vi "בדיקת זמן מיתוג הממסר 6.vi"(8 "error":errorcluster, 11 "Path for Log":path) -> (0 "error out":errorcluster, 1 "בטוח כן/לא":bool, 2 "בדיקת זמן מיתוג הממסר":dbl, 7 "Userresult":bool)   [LabVIEW 2014]
uses:
  <instrlib>/niDMM/nidmm.llb/niDMM Function.ctl
  <instrlib>/niDMM/nidmm.llb/niDMM Resolution in Digits.ctl
  <vilib>/DAQmx/create/channels.llb/DAQmx Create Channel (DO-Digital Output).vi
  <instrlib>/niDMM/nidmm.llb/niDMM Configure Measurement Digits.vi
  <vilib>/DAQmx/write.llb/DAQmx Write (Digital Bool 1Line 1Point).vi
panel:
  in  "התחל":bool
  # "Right-Click to\nexplain error"
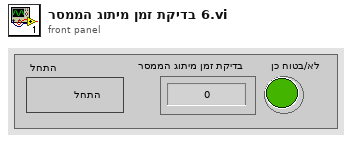
[diagram p1: front panel]
types:
  T1 = enum32{"Invalid", "Standard", "Closed", "Hidden", "Minimized", "Maximized"}
  T2 = typedef "niDMM Function.ctl" = enum16{"DC Volts", "AC Volts", "DC Current", "AC Current", "2-wire Resistance", "4-wire Resistance", "Diode", "Frequency", "Period", "AC Volts DC Coupled", "Capacitance", "Inductance", "Temperature"}
  T3 = typedef "niDMM Resolution in Digits.ctl" = dbl
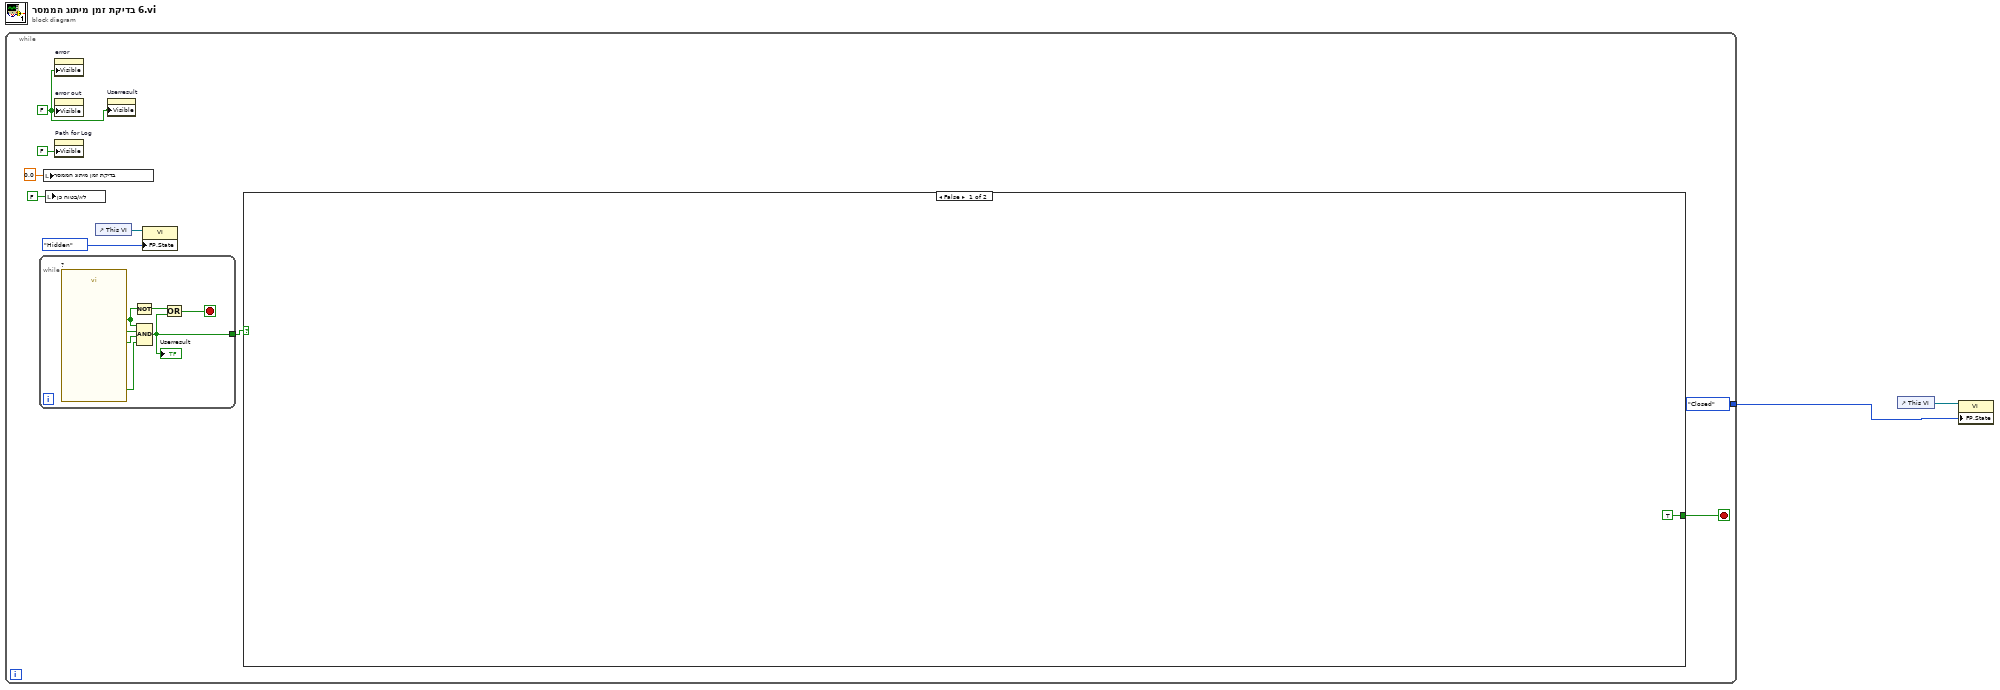
[diagram p0: block diagram]
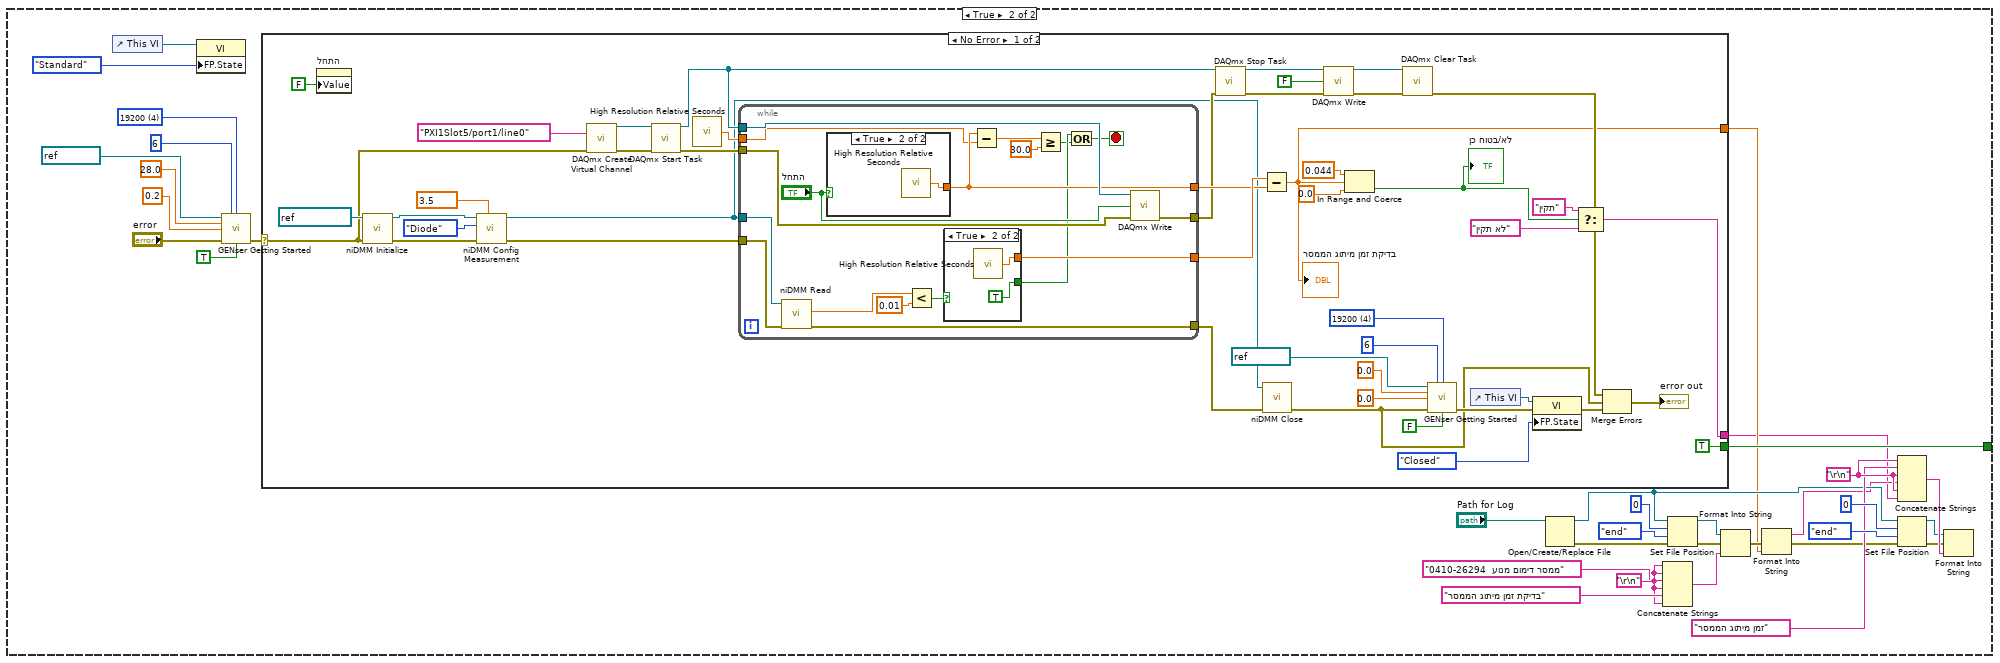
[diagram p2: hidden frame]
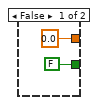
[diagram p3: hidden frame]
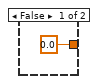
[diagram p4: hidden frame]
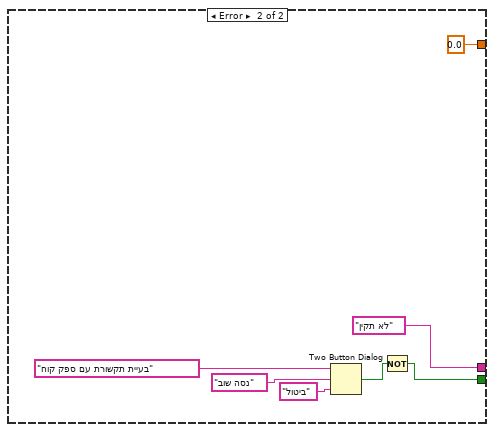
[diagram p5: hidden frame]
diagram:
  n1 = while {
    tunnel: [T1."Closed" ("Front Panel Window:State")] -> w1
    stop <- w4 stop-if-true
    w5 = FALSE ("Visible")
    n2 = while {
      tunnel: [w12] -> w9
      stop <- w15 stop-if-true
      n3 = call "?"() -> ("הדקי הרב מודד"=w16:bool, "(מגע שלילי (מעטפת"=w17:bool, "C מגע חיובי"=w18:bool, "OK"=w13:bool)  [unwired: 15 in, 1 out]
      n4 = Not(x=w13) -> (.not. x?=w14:bool)
      n5 = Compound Arithmetic op=AND(w13, w18, w17, w16) -> (w12:bool)
      "Userresult" <- w12
      n6 = Or(x=w14, y=w12) -> (x .or. y?=w15:bool)
    }
    n7 = local write "בדיקת זמן מיתוג הממסר"(0.0 ("בדיקת זמן מיתוג הממסר")) -> ()
    n8 = local write "בטוח כן/לא"(FALSE ("בטוח כן/לא")) -> ()
    n9 = property on="error" class="Clust (strict)"("Visible"=w5) -> ()  [unwired: 2 in, 2 out]
    n10 = property on="error out" class="Clust (strict)"("Visible"=w5) -> ()  [unwired: 2 in, 2 out]
    n11 = property on="Path for Log" class="Path"("Visible"=FALSE) -> ()  [unwired: 2 in, 2 out]
    n12 = control-ref of="This VI"() -> (w11:refnum<vi>)
    n13 = property on="Userresult" class="Bool (strict)"("Visible"=w5) -> ()  [unwired: 2 in, 2 out]
    n14 = property class="VI"(reference=w11, "FP.State"=T1."Hidden" ("Front Panel Window:State")) -> ()  [unwired: 1 in, 2 out]
    n15 = case shown="False" w9 {
      tunnel: [TRUE ("T button?") w46] -> w4
      frame False {
      }
      frame True {
        w30 = "\r\n"
        w37 = "\r\n"
        w49 = u16 4 items=["1200", "2400", "4800", "9600", "19200"] ("BAUD")
        n16 = control-ref of="This VI"() -> (w45:refnum<vi>)
        n17 = property class="VI"(reference=w45, "FP.State"=T1."Standard" ("Front Panel Window:State")) -> ()  [unwired: 1 in, 2 out]
        n18 = call "GENser Getting Started.vi"("VISA"=refnum<visa-resource-name> "COM6", "GEN Addr"=i16 6, "BAUD"=w49, "Voltage Limit"=28.0, "Current Limit"=0.2, "error"="error", "Output On (T)"=TRUE) -> ("error out"=w51:errorcluster)  [unwired: 5 in, 3 out]
        n19 = case shown="No Error" w51 {
          selector: w51 -> [w55 _]
          tunnel: [TRUE ("T button?") w123] -> w46
          tunnel: [w73 0.0] -> w22
          tunnel: [w69 "לא תקין"] -> w21
          frame No Error {
            w61 = T3 3.5 items=["3 1/2"=3.5, "4 1/2"=4.5, "5 1/2"=5.5, "6 1/2"=6.5, "7 1/2"=7.5] ("Resolution in Digits")
            w92 = u16 4 items=["1200", "2400", "4800", "9600", "19200"] ("BAUD")
            n20 = property on="התחל" class="Bool (strict)"("Value"=FALSE ("data")) -> ()  [unwired: 2 in, 2 out]
            n21 = call <instrlib>:"niDMM Initialize.vi"("error in (no error)"=w55, "Instrument Descriptor"=refnum<k15> "PXI1Slot9") -> ("error out"=w59:errorcluster, "instrument handle out"=w60:refnum<k15>)  [unwired: 8 in]
            n22 = call-poly <instrlib>:"niDMM Config Measurement.vi"("Resolution in Digits"=w61, "error in (no error)"=w59, "Function"=niDMM_Function."Diode", "instrument handle"=w60) -> ("error out"=w58:errorcluster, "instrument handle out"=w56:refnum<k15>)  [unwired: 6 in]
            n23 = call-poly <vilib>:"DAQmx Create Virtual Channel.vi"("lines"=tag "PXI1Slot5/port1/line0", "error in"=w55) -> ("task out"=w66:refnum<k21>, "error out"=w67:errorcluster)  [unwired: 12 in]
            n24 = call <vilib>:"DAQmx Start Task.vi"("task/channels in"=w66, "error in"=w67) -> ("task out"=w57:refnum<k21>, "error out"=w64:errorcluster)  [unwired: 12 in]
            n25 = call <vilib>:"High Resolution Relative Seconds.vi"() -> ("relative seconds"=w63:dbl)
            n26 = while {
              tunnel: [w108] -> w81
              tunnel: [w116] -> w82
              tunnel: [w115] -> w80
              tunnel: [w110] -> w79
              tunnel: w57 -> [w114]
              tunnel: w64 -> [w113]
              tunnel: w63 -> [w107]
              tunnel: w58 -> [w100]
              tunnel: w56 -> [w99]
              stop <- w104 stop-if-true
              n27 = call <instrlib>:"niDMM Read.vi"("error in (no error)"=w100, "instrument handle"=w99) -> ("error out"=w110:errorcluster, "Measurement"=w112:dbl)  [unwired: 7 in, 1 out]
              n28 = case shown="True" "התחל" {
                tunnel: [0.0 ("relative seconds") w122] -> w108
                frame False {
                }
                frame True {
                  n29 = call <vilib>:"High Resolution Relative Seconds.vi"() -> ("relative seconds"=w122:dbl)
                }
              }
              n30 = Less?(x=w112, y=0.01) -> (x < y?=w101:bool)
              n31 = case shown="True" w101 {
                tunnel: [0.0 ("relative seconds") w120] -> w116
                tunnel: [FALSE TRUE] -> w103
                frame False {
                }
                frame True {
                  n32 = call <vilib>:"High Resolution Relative Seconds.vi"() -> ("relative seconds"=w120:dbl)
                }
              }
              n33 = Subtract(x=w108, y=w107) -> (x-y=w106:dbl)
              n34 = Greater Or Equal?(x=w106, y=30.0) -> (x >= y?=w102:bool)
              n35 = Or(x=w103, y=w102) -> (x .or. y?=w104:bool)
              n36 = call-poly <vilib>:"DAQmx Write.vi"("task/channels in"=w114, "data"="התחל", "error in"=w113) -> ("error out"=w115:errorcluster)  [unwired: 10 in, 2 out]
            }
            n37 = call <vilib>:"DAQmx Stop Task.vi"("task/channels in"=w57, "error in"=w80) -> ("task out"=w87:refnum<k21>, "error out"=w86:errorcluster)  [unwired: 12 in]
            n38 = Subtract(x=w82, y=w81) -> (x-y=w73:dbl)
            "בדיקת זמן מיתוג הממסר" <- w73
            n39 = call <instrlib>:"niDMM Close.vi"("error in (no error)"=w79, "instrument handle"=w56) -> ("error out"=w54:errorcluster)  [unwired: 9 in]
            n40 = call-poly <vilib>:"DAQmx Write.vi"("task/channels in"=w87, "data"=FALSE, "error in"=w86) -> ("task out"=w84:refnum<k21>, "error out"=w85:errorcluster)  [unwired: 10 in, 1 out]
            n41 = In Range and Coerce(upper limit=0.044, x=w73, lower limit=0.0) -> (In Range?=w70:bool)  [unwired: 1 out]
            "בטוח כן/לא" <- w70
            n42 = call <vilib>:"DAQmx Clear Task.vi"("task in"=w84, "error in"=w85) -> ("error out"=w77:errorcluster)  [unwired: 13 in]
            n43 = call "GENser Getting Started.vi"("VISA"=refnum<visa-resource-name> "COM6", "GEN Addr"=i16 6, "BAUD"=w92, "Voltage Limit"=0.0, "Current Limit"=0.0, "error"=w54, "Output On (T)"=FALSE) -> ("error out"=w91:errorcluster)  [unwired: 5 in, 3 out]
            n44 = control-ref of="This VI"() -> (w90:refnum<vi>)
            n45 = property class="VI"(reference=w90, error in=w91, "FP.State"=T1."Closed" ("Front Panel Window:State")) -> (error out=w76:errorcluster)  [unwired: 1 out]
            n46 = Select(t="תקין", s=w70, f="לא תקין") -> (s? t:f=w69:string)
            n47 = Merge Errors(w77, w54, w76) -> (→"error out":errorcluster)
          }
          frame Error {
            n48 = Two Button Dialog(message="בעיית תקשורת עם ספק קוח", 1:"ביטול" ("F button name (\"Cancel\")"), 2:"נסה שוב" ("T button name (\"OK\")")) -> (T button?=w124:bool)
            n49 = Not(x=w124) -> (.not. x?=w123:bool)
          }
        }
        n50 = Open/Create/Replace File(file path (use dialog)="Path for Log") -> (refnum out=w26:refnum<file>, error out=w27:errorcluster)  [unwired: 5 in, 1 out]
        n51 = Concatenate Strings(w37, w37, "0410-26294  ממסר דימום מנוע", w37, "בדיקת זמן מיתוג הממסר", w37) -> (w40:string)
        n52 = Set File Position(offset (in bytes) (0)=i64 0, refnum=w26, from (0:start)=enum16{"start", "end", "current"}."end", error in=w27) -> (refnum out=w38:refnum<file>, error out=w36:errorcluster)
        n53 = Format Into String(initial string=w38, error in=w36, w40) -> (error out=w25:errorcluster)  [unwired: 1 in, 1 out]
        n54 = Format Into String(error in=w25, w22) -> (resulting string=w23:string, error out=w24:errorcluster)  [unwired: 2 in]
        n55 = Concatenate Strings(w30, "זמן מיתוג הממסר", w30, w23, w30, w21) -> (w35:string)
        n56 = Set File Position(offset (in bytes) (0)=i64 0, refnum=w26, from (0:start)=enum16{"start", "end", "current"}."end", error in=w24) -> (refnum out=w33:refnum<file>, error out=w34:errorcluster)
        n57 = Format Into String(initial string=w33, error in=w34, w35) -> ()  [unwired: 1 in, 2 out]
      }
    }
  }
  n58 = control-ref of="This VI"() -> (w2:refnum<vi>)
  n59 = property class="VI"(reference=w2, "FP.State"=w1) -> ()  [unwired: 1 in, 2 out]
